vi "UploadKVPair.vi"(8 "error in":errorcluster, 11 "Payload":string) -> (0 "error out":errorcluster, 1 "headers":string="HTTP/1.1 200 OK\r\nDate: Wed, 20 Nov 2024 13:14:40 GMT\r\nContent-Type: text/plain;charset=UTF-8\r\nContent-Length: 24\r\nConnection: keep-alive\r\nReport-To: {\"endpoints\":[{\"url\":\"https:\\/\\/a.nel.cloudflare.com\\/report\\/v4?s=mEqVRT0JaB8UfpwofkBtcUolZEfBLjG29cm9RyWkolcXw0PhDwccmong3dq0mG3tSZbWaPLkwwkhpz5o4mjk59hYimhsQFYsFkHnAQBUd1ZE%2FSfzdwAI4ES6sLWtbA6EjjJFWIBeflTkrcoIgUySxGul6EZ7Iao0Pfg0FWbpZkFo8A%3D%3D\"}],\"group\":\"cf-nel\",\"max_age\":604800}\r\nNEL: {\"success_fraction\":0,\"report_to\":\"cf-nel\",\"max_age\":604800}\r\nServer: cloudflare\r\nCF-RAY: 8e58b4521aa856c9-OSL\r\nalt-svc: h3=\":443\"; ma=86400\r\nserver-timing: cfL4;desc=\"?proto=TCP&rtt=20047&sent=5&recv=7&lost=0&retrans=0&sent_bytes=2873&recv_bytes=869&delivery_rate=197253&cwnd=252&unsent_bytes=0&cid=e8c4a2d6051ff16b&ts=348&x=0\"\r\n\r\n", 2 "body":string="Data stored successfully")   [LabVIEW 2024]
uses:
  <vilib>/httpClient/POSTBuffer.vi
  <vilib>/httpClient/LabVIEWHTTPClient.lvlib
panel:
  in  "header":string(combo)="Content-Type"
  in  "value":string="application/json"
  in  "url":string="https://payload-data.viaslavdem.workers.dev"
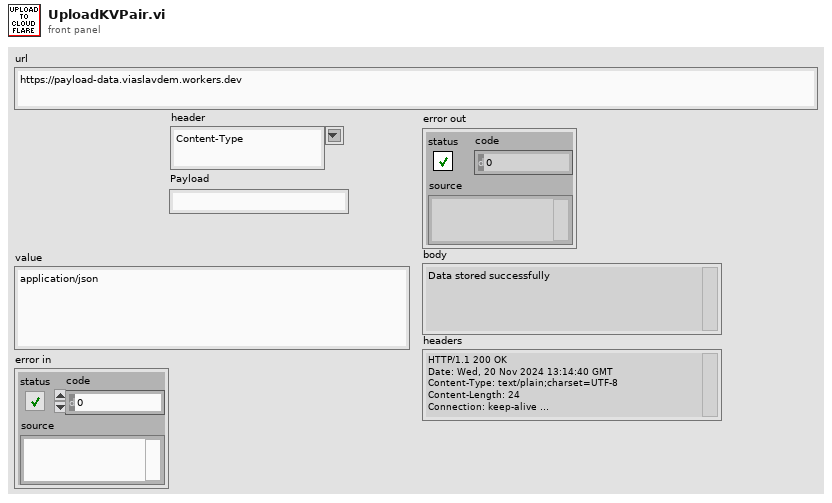
[diagram p1: front panel]
types:
  T1 = typedef "LabVIEWHTTPClient.lvlib/ClientHandle.ctl" = refnum<k1>
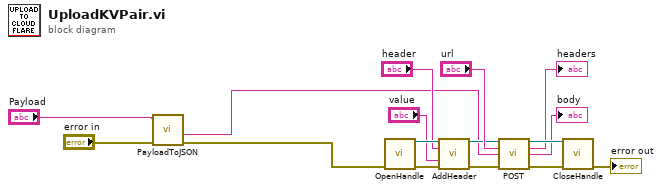
[diagram p0: block diagram]
diagram:
  n1 = call "PayloadToJSON.vi"("error in"="error in", "Payload"="Payload") -> ("error out"=w2:errorcluster, "JSON string"=w3:string)  [unwired: 6 in, 2 out]
  n2 = call <vilib>:"OpenHandle.vi"("error in (no error)"=w2) -> ("client handle out"=w13:T1, "error out"=w12:errorcluster)  [unwired: 13 in]
  n3 = call <vilib>:"AddHeader.vi"("client handle"=w13, "header"="header", "value"="value", "error in (no error)"=w12) -> ("client handle out"=w5:T1, "error out"=w11:errorcluster)  [unwired: 10 in]
  n4 = call-poly <vilib>:"POST.vi"("client handle"=w5, "url"="url", "buffer"=w3, "error in (no error)"=w11) -> ("client handle out"=w16:T1, "headers"=→"headers":string, "body"=→"body":string, "error out"=w15:errorcluster)  [unwired: 8 in]
  n5 = call <vilib>:"CloseHandle.vi"("client handle"=w16, "error in (no error)"=w15) -> ("error out"=→"error out":errorcluster)  [unwired: 13 in]
